vi "VIQA String Selection.vi"(8 "error in (no error)":errorcluster, 9 "PlatMods":T1, 10 "Char":i16, 11 "String in":refnum<vi>) -> (0 "error out":errorcluster, 3 "Discard":bool)   [LabVIEW 2018, in "VI Quality.lvlib"]
doc: "This VI manipulates the VI description string for bold (ctrl-b) or select all (ctrl-a) functions."
uses:
  VI Quality.lvlib
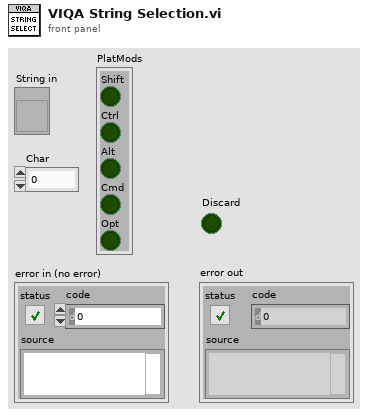
[diagram p1: front panel]
types:
  T1 = cluster{"Shift":bool, "Ctrl":bool, "Alt":bool, "Cmd":bool, "Opt":bool}
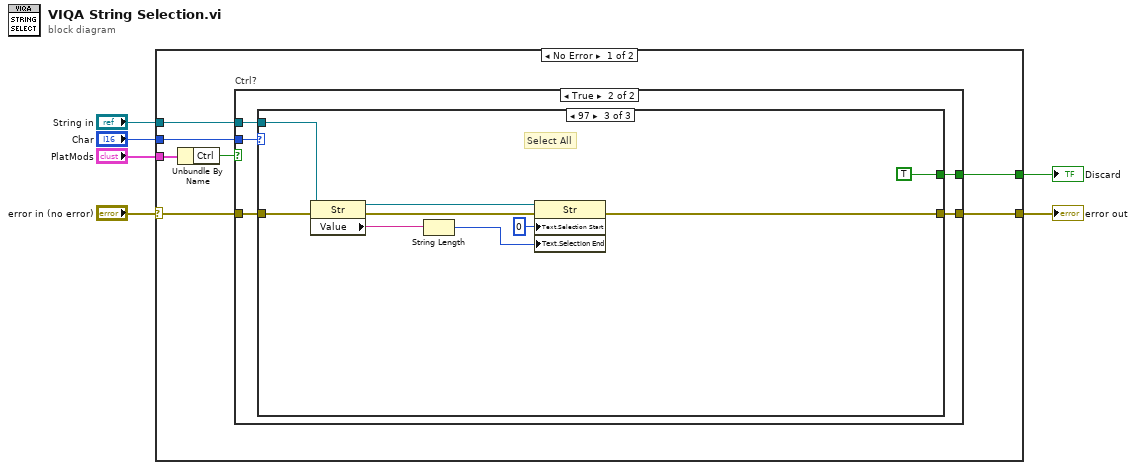
[diagram p0: block diagram]
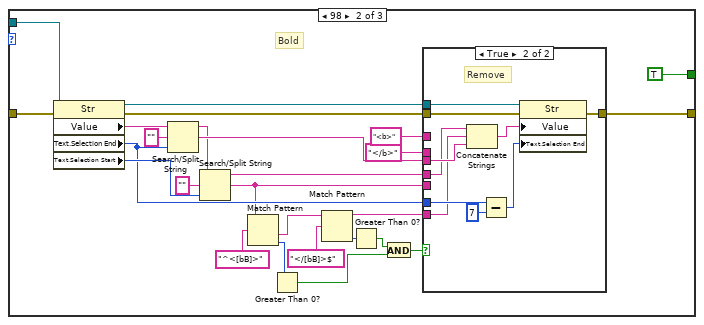
[diagram p4: hidden frame]
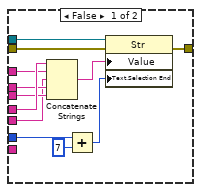
[diagram p5: hidden frame]
diagram:
  n1 = case shown="No Error" "error in (no error)" {
    selector: "error in (no error)" -> [w10 w78]
    tunnel: [w13 _] -> w6
    tunnel: "Char" -> [w12 _]
    tunnel: [w11 w78] -> w4
    tunnel: "String in" -> [w9 _]
    tunnel: "PlatMods" -> [w8 _]
    frame No Error {
      n2 = Unbundle By Name(w8) -> ("Ctrl"=w7:bool)
      n3 = case "Ctrl?" shown="True" w7 {
        tunnel: w9 -> [_ w19]
        tunnel: w10 -> [w14 w18]
        tunnel: [w14 w17] -> w11
        tunnel: w12 -> [_ w16]
        tunnel: [_ w15] -> w13
        frame False {
        }
        frame True {
          n4 = case shown="97" w16 {
            tunnel: w19 -> [_ w46 w77]
            tunnel: w18 -> [w20 w43 w76]
            tunnel: [w20 w40 w73] -> w17
            tunnel: [_ TRUE TRUE] -> w15
            frame 0, Default {
            }
            frame 98 {
              # "Bold"
              n5 = property class="Str"(reference=w46, error in=w43) -> (reference out=w41:refnum<vi>, error out=w42:errorcluster, "Value"=w44:string, "Text.Selection End"=w33:u32, "Text.Selection Start"=w38:u32)
              n6 = Search/Split String(string=w44, search string/char (-)="", offset (0)=w33) -> (substring before match=w30:string, match + rest of string=w34:string)  [unwired: 1 out]
              n7 = Search/Split String(string=w30, search string/char (-)="", offset (0)=w38) -> (substring before match=w37:string, match + rest of string=w21:string)  [unwired: 1 out]
              n8 = Match Pattern(string=w21, regular expression="^<[bB]>") -> (after substring=w22:string, offset past match=w27:i32)  [unwired: 1 in, 2 out]
              n9 = Greater Than 0?(x=w27) -> (x > 0?=w25:bool)
              n10 = Match Pattern(string=w22, regular expression="</[bB]>$") -> (before substring=w23:string, offset past match=w28:i32)  [unwired: 1 in, 2 out]
              n11 = Greater Than 0?(x=w28) -> (x > 0?=w26:bool)
              n12 = And(x=w26, y=w25) -> (x .and. y?=w24:bool)
              n13 = case shown="True" w24 {
                tunnel: w42 -> [w58 w68]
                tunnel: w41 -> [w57 w67]
                tunnel: [w56 w66] -> w40
                tunnel: w37 -> [w55 w60]
                tunnel: "<b>" ("string") -> [w54 _]
                tunnel: "</b>" ("string") -> [w53 _]
                tunnel: w34 -> [w52 w61]
                tunnel: w33 -> [w50 w64]
                tunnel: w21 -> [w47 _]
                tunnel: w23 -> [_ w59]
                frame False {
                  n14 = Concatenate Strings(w55, w54, w47, w53, w52) -> (w51:string)
                  n15 = Add(x=w50, y=u32 7) -> (x+y=w48:u32)
                  n16 = property class="Str"(reference=w57, error in=w58, "Value"=w51, "Text.Selection End"=w48) -> (error out=w56:errorcluster)  [unwired: 1 out]
                }
                frame True {
                  # "Remove"
                  n17 = Concatenate Strings(w60, w59, w61) -> (w65:string)
                  n18 = Subtract(x=w64, y=u32 7) -> (x-y=w62:u32)
                  n19 = property class="Str"(reference=w67, error in=w68, "Value"=w65, "Text.Selection End"=w62) -> (error out=w66:errorcluster)  [unwired: 1 out]
                }
              }
            }
            frame 97 {
              # "Select All"
              n20 = property class="Str"(reference=w77, error in=w76) -> (reference out=w74:refnum<vi>, error out=w75:errorcluster, "Value"=w71:string)
              n21 = String Length(string=w71) -> (length=w69:i32)
              n22 = property class="Str"(reference=w74, error in=w75, "Text.Selection Start"=u32 0 ("Text.Selection:Start"), "Text.Selection End"=w69) -> (error out=w73:errorcluster)  [unwired: 1 out]
            }
          }
        }
      }
    }
    frame Error {
    }
  }
  "Discard" <- w6
  "error out" <- w4
